vi "tensão da bateria (SubVI).vi"(11 "data in":string) -> (3 "Numeric":dbl)   [LabVIEW 2015]
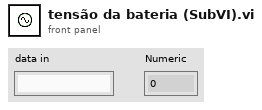
[diagram p1: front panel]
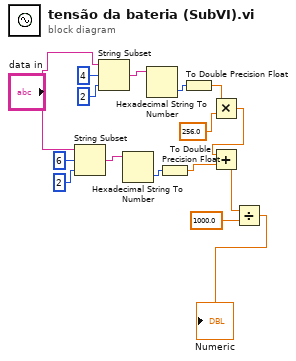
[diagram p0: block diagram]
diagram:
  n1 = String Subset(string="data in", offset (0)=6, length (rest)=2 ("length (rest)")) -> (substring=w9:string)
  n2 = String Subset(string="data in", offset (0)=4, length (rest)=2 ("length (rest)")) -> (substring=w3:string)
  n3 = Hexadecimal String To Number(string=w9) -> (number=w5:u32)  [unwired: 2 in, 1 out]
  n4 = Hexadecimal String To Number(string=w3) -> (number=w4:u32)  [unwired: 2 in, 1 out]
  n5 = To Double Precision Float(number=w5) -> (double precision float=w11:dbl)
  n6 = To Double Precision Float(number=w4) -> (double precision float=w10:dbl)
  n7 = Multiply(x=w10, y=256.0) -> (x*y=w12:dbl)
  n8 = Add(x=w12, y=w11) -> (x+y=w15:dbl)
  n9 = Divide(x=w15, y=1000.0) -> (x/y=→"Numeric":dbl)
